vi "TSM SSC Digital Filter Sites.vi"(0 "Digital TSM In":T1, 5 "Desired Sites":i32[](array[numeric])) -> (4 "Digital TSM Out":T1)   [LabVIEW 2020]
doc: "Use this VI to filter the Digital Cluster to contain only sessions and information pertaining to the desired sites. Note that the cluster information output by this function may be used for instrument control but should NOT be used to publish data to TSM."
uses:
  TSM SSC Digital.ctl
  <vilib>/NI_TestStand_SemiconductorModule/NI_TestStand_Semiconductor_Module.lvlibp/PinMap/Digital Pattern/PinQueryContext/DigitalPatternPinQueryContext.lvclass
  SSC Digital/SSC Digital.ctl
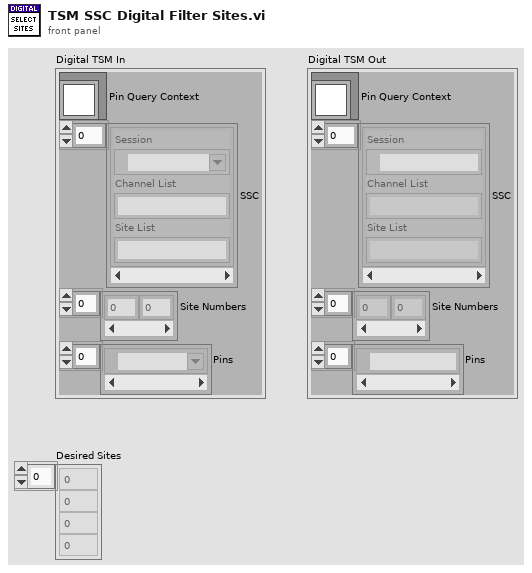
[diagram p1: front panel]
types:
  T1 = typedef "TSM SSC Digital.ctl" = cluster{"Pin Query Context":refnum<class "DigitalPatternPinQueryContext.lvclass">, "SSC":T2[], "Site Numbers":i32[], "Pins":tag[]}
  T2 = typedef "SSC Digital.ctl" = cluster{"Session":refnum<k15>, "Channel List":string, "Site List":string}
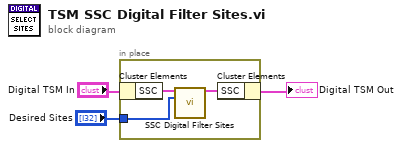
[diagram p0: block diagram]
diagram:
  n1 = in-place {
    in-place-border: "Desired Sites" -> [w6]
    n2 = in-place-cluster #1("Digital TSM In") -> ("SSC"=w5:T2[])
    n3 = call "SSC Digital Filter Sites.vi"("Digital SSC In"=w5, "Desired Sites"=w6) -> ("Digital SSC Out with requested sites"=w4:T2[])  [unwired: 13 in]
    n4 = in-place-cluster #1("SSC"=w4) -> (→"Digital TSM Out":T1)
  }
